vi "Read Digital Outputs.vi"(8 "error in (no error)":errorcluster, 11 "PXI6521 in":refnum<class "PXI6521.lvclass">) -> (0 "error out":errorcluster, 3 "PXI6521 out":refnum<class "PXI6521.lvclass">)   [LabVIEW 2018, in "PXI6521.lvlib" / "PXI6521.lvclass"]
uses:
  PXI6521.lvclass
  PPLs/DigitalIO/Parent/DigitalIO.lvlibp/DigitalIO.lvclass
  C:/Projects/LabVIEW/PPLs/DigitalIO/Parent/DigitalIO.lvlibp/DigitalIO.lvclass
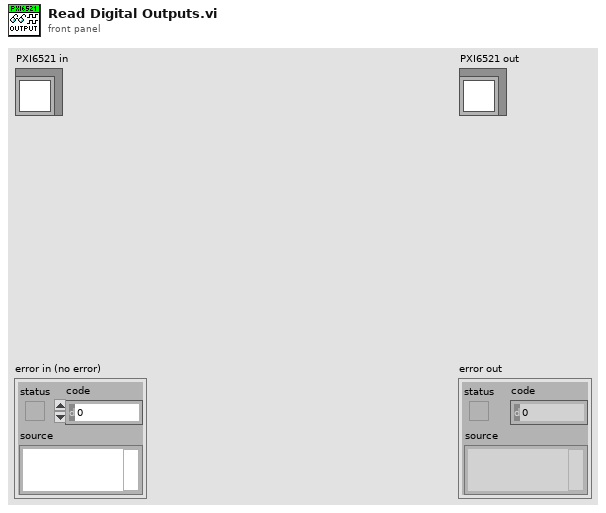
[diagram p1: front panel]
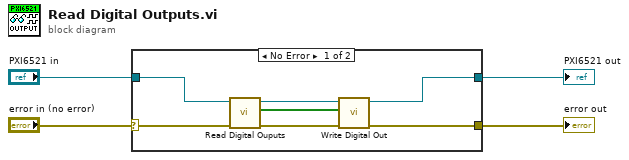
[diagram p0: block diagram]
diagram:
  n1 = case shown="No Error" "error in (no error)" {
    selector: "error in (no error)" -> [w10 w12]
    tunnel: "PXI6521 in" -> [w11 w13]
    tunnel: [w6 w12] -> w2
    tunnel: [w5 w13] -> w1
    frame No Error {
      n2 = call "Read Digital Ouputs.vi"("error in (no error)"=w10, "PXI6521 in"=w11) -> ("error out"=w7:errorcluster, "Digital Outputs Status"=w8:bool[], "PXI6521 out"=w9:refnum<class "PXI6521.lvclass">)  [unwired: 7 in]
      n3 = call "Write Digital Out.vi"("error in (no error)"=w7, "Digital Out"=w8, "DigitalIO in"=w9) -> ("error out"=w6:errorcluster, "DigitalIO out"=w5:refnum<class "PXI6521.lvclass">)  [unwired: 7 in]
    }
    frame Error {
    }
  }
  "error out" <- w2
  "PXI6521 out" <- w1
